vi "PH_Tektronix_7000.check Error.vi"(0 "i ref in":refnum<vi>, 5 "error in":errorcluster) -> (14 "i ref out":refnum<vi>, 19 "error out":errorcluster)   [LabVIEW 2014, in "PH_Tektronix_7000.lvlib"]
doc: "This VI has to be set after any communication with the hardware: It sets the busy flag depending on the hardware error (which is queried) to false or failure; the hardware error is indicated at the GUI element (tip strip).This VI is the counterpart to \"start communication\"."
uses:
  PH_Tektronix_7000.lvlib
  PH_Basics/PH_StatusHandler/PH_StatusHandler.Status.ctl
  PH_Basics/PH_Common/PH_Common.lvlib
  instr.lib/Tektronix7000Series/Tektronix 7000 Series - Driver np.lvlib
  PH_Basics/PH_StatusHandler/PH_StatusHandler.lvlib
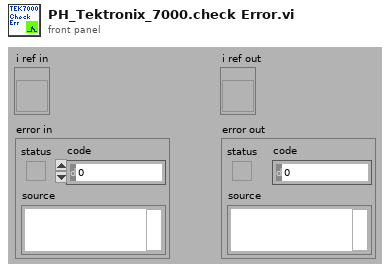
[diagram p1: front panel]
types:
  T1 = typedef "PH_Tektronix_7000.lvlib/PH_Tektronix_7000.i attribute.ctl" = cluster{"VISA Resource Name":refnum<visa-resource-name>, "IDN":cluster{"Instrument Driver":string, "Instrument Firmware":string, "Model":string, "Serial Number":string}, "Selftest":cluster{"Result":i32, "Message":string}, "Trigger Configuration":T2, "Acquisition Configuration":T3, "GUI Refs":T4, "State":T5, "Error Message":string, "Allow Prdc Loop?":bool, "Channel 1":T6, "Channel 2":T6, "Channel 3":T6, "Channel 4":T6, "Data CH 1":waveform(dbl), "Data CH 2":waveform(dbl), "Data CH 3":waveform(dbl), "Data CH 4":waveform(dbl), "Allow config?":bool, "Name Channel 1":string, "Name Channel 2":string, "Name Channel 3":string, "Name Channel 4":string, "Fetch Data before sending to PSDB?":bool, "Constructor passed?":bool, "Data taken at":timestamp, "Plot Colors":u32[], "Default VISA Resource":string}
  T2 = typedef "PH_Tektronix_7000.lvlib/PH_Tektronix_7000.Trigger Config.ctl" = cluster{"Source":u16, "Level [V]":dbl, "Slope":u16, "Coupling":u16, "Trigger Mode":u16}
  T3 = typedef "PH_Tektronix_7000.lvlib/PH_Tektronix_7000.Acquisition Config.ctl" = cluster{"Record Length":u32, "Timebase [s/div]":dbl, "Position [%]":dbl, "Acquisition Type":u16, "Average Waveforms":i32, "Envelope Waveforms":i32, "WfmDB Samples":i32, "Continuous?":bool, "Delay [s]":dbl, "Run?":bool}
  T4 = typedef "PH_Tektronix_7000.lvlib/PH_Tektronix_7000.GUI Refs.ctl" = cluster{"Graph":refnum<vi>, "State":refnum<vi>, "Delete":refnum<vi>, "VISA Resource":refnum<vi>, "Allow Configure":refnum<vi>, "Fetch Data":refnum<vi>, "Fetch before sending Data to PSDB":refnum<vi>, "Name Channel 1":refnum<vi>, "Name Channel 2":refnum<vi>, "Name Channel 3":refnum<vi>, "Name Channel 4":refnum<vi>, "Prdc Intervall [ms]":refnum<vi>, "Data taken":refnum<vi>, "Model":refnum<vi>, "Serial Number":refnum<vi>, "Firmware":refnum<vi>, "Driver":refnum<vi>, "Acquisition":refnum<vi>, "Trigger":refnum<vi>, "Cursor: D Time [s]":refnum<vi>, "Cursor: D Signal [V]":refnum<vi>, "Channel 1":refnum<vi>, "Channel 2":refnum<vi>, "Channel 3":refnum<vi>, "Channel 4":refnum<vi>}
  T5 = typedef "PH_StatusHandler.lvlib/PH_StatusHandler.Status.ctl" = i16
  T6 = typedef "PH_Tektronix_7000.lvlib/PH_Tektronix_7000.Channel Config.ctl" = cluster{"Enable Channel":bool, "Bandwidth":u16, "Input Impedance":u16, "Vertical Coupling":u16, "Probe Attenuation":dbl, "Range [V/div]":dbl, "Position [div]":dbl, "Bandwidth raw":string}
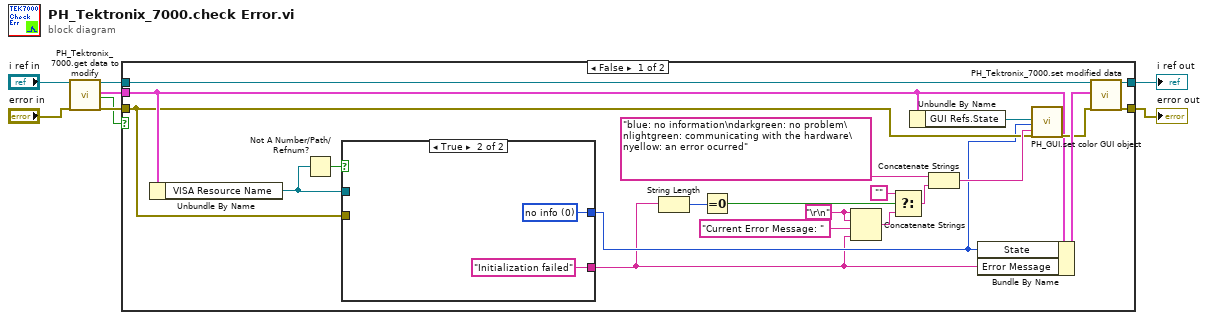
[diagram p0: block diagram]
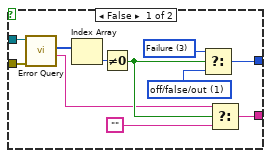
[diagram p2: hidden frame]
diagram:
  n1 = call "PH_Tektronix_7000.get data to modify.vi"("i ref in"="i ref in", "error in (no error)"="error in") -> ("i ref out"=w2:refnum<vi>, "i attribute"=w4:T1, "timed out"=w1:bool, "error out"=w3:errorcluster)  [unwired: 14 in]
  n2 = case shown="False" w1 {
    tunnel: [w29 w43] -> w8
    tunnel: w3 -> [w13 w43]
    tunnel: w2 -> [w28 w44]
    tunnel: [w27 w44] -> w6
    tunnel: w4 -> [w14 _]
    frame False {
      w18 = "\r\n"
      n3 = Unbundle By Name(w14) -> ("VISA Resource Name"=w10:refnum<visa-resource-name>)
      n4 = Not A Number/Path/Refnum?(number/path/refnum=w10) -> (NaN/Path/Refnum?=w9:bool)
      n5 = case shown="True" w9 {
        tunnel: w13 -> [w40 _]
        tunnel: [w34 w42] -> w12
        tunnel: [w31 "Initialization failed" ("Error Message")] -> w11
        tunnel: w10 -> [w30 _]
        frame False {
          w37 = T5 1 items=["no info", "off/false/out", "on/true/in", "Failure", "Alarm", "Status 1", "Status 2", "Status 3"] ("f")
          w38 = T5 3 items=["no info", "off/false/out", "on/true/in", "Failure", "Alarm", "Status 1", "Status 2", "Status 3"] ("State")
          n6 = call "Error Query.vi"("error in (no error)"=w40, "VISA resource name"=w30) -> ("Error Message"=w33:string, "Error Code"=w35:i32[])  [unwired: 6 in, 2 out]
          n7 = Index Array(array=w35) -> (element=w39:i32)  [unwired: 1 in]
          n8 = Not Equal To 0?(x=w39) -> (x != 0?=w36:bool)
          n9 = Select(t=w38, s=w36, f=w37) -> (s? t:f=w34:T5)
          n10 = Select(t=w33, s=w36, f="") -> (s? t:f=w31:string)
        }
        frame True {
          w42 = T5 0 items=["no info", "off/false/out", "on/true/in", "Failure", "Alarm", "Status 1", "Status 2", "Status 3"] ("f")
        }
      }
      n11 = String Length(string=w11) -> (length=w21:i32)
      n12 = Equal To 0?(x=w21) -> (x = 0?=w20:bool)
      n13 = Concatenate Strings(w18, w18, "Current Error Message: " ("string"), w11) -> (w16:string)
      n14 = Select(t="", s=w20, f=w16) -> (s? t:f=w15:string)
      n15 = Unbundle By Name(w14) -> ("GUI Refs.State"=w24:refnum<vi>)
      n16 = Concatenate Strings("blue: no information\ndarkgreen: no problem\nlightgreen: communicating with the hardware\nyellow: an error ocurred", w15) -> (w22:string)
      n17 = Bundle By Name(cluster=w14, "State"=w12, "Error Message"=w11) -> (w26:T1)
      n18 = call "PH_GUI.set color GUI object.vi"("GUI object Ref"=w24, "State"=w12, "error in (no error)"=w13, "Tip Strip (N/A)"=w22) -> ("error out"=w25:errorcluster)  [unwired: 15 in]
      n19 = call "PH_Tektronix_7000.set modified data.vi"("i ref in"=w28, "i attribute"=w26, "error in (no error)"=w25) -> ("i ref out"=w27:refnum<vi>, "error out"=w29:errorcluster)  [unwired: 15 in]
    }
    frame True {
    }
  }
  "error out" <- w8
  "i ref out" <- w6
